vi "OverlayArcCenterSize.vi"(0 "Image Reference In":T3, 1 "GroupName":string, 2 "Start Angle (degrees)":dbl format="%.2f", 3 "End Angle (degrees)":dbl format="%.2f", 5 "Center-Point":T1, 7 "Size":T1, 11 "error in":errorcluster, 12 "Drawing Mode (Fill)":T2=enum."Fill", 13 "Color":u32(colorbox)=16711680) -> (4 "Image Reference Out":T3, 15 "error out":errorcluster)   [LabVIEW 2024, in "OpenLvVision_Overlays.lvlib"]
doc: "Overlay a arc on top of an image.\nDraws the arc arround a center point."
uses:
  OpenLvVision_Overlays.lvlib
  <vilib>/OpenLvVision/OpenLvVision_Image/Management/TypeDef/OLV Image.ctl
  TypeDefs/DrawingMode.ctl
  TypeDefs/PointI32.ctl
  <vilib>/OpenLvVision/OpenLvVision_Image/Management/OLV Management.lvlib
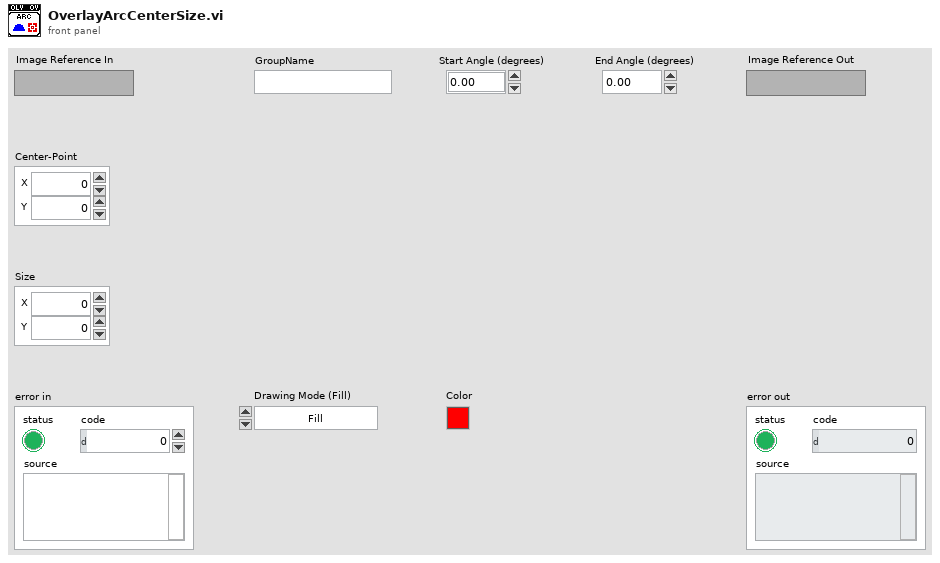
[diagram p1: front panel]
types:
  T1 = typedef "OpenLvVision_Overlays.lvlib/PointI32.ctl" = cluster{"X":i32, "Y":i32}
  T2 = typedef "OpenLvVision_Overlays.lvlib/DrawingMode.ctl" = enum16{"Frame", "Fill"}
  T3 = typedef "OLV OpenLvVision_Image.lvlib/OLV Management.lvlib/OLV Image.ctl" = refnum<image>
  T4 = typedef "OLV OpenLvVision_Image.lvlib/OLV DataAccess.lvlib/OLV RectangleI32.ctl" = cluster{"Left":i32, "Top":i32, "Right":i32, "Bottom":i32}
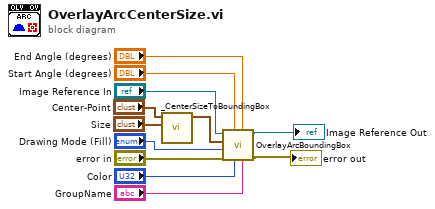
[diagram p0: block diagram]
diagram:
  n1 = call "_CenterSizeToBoundingBox.vi"("Size"="Size", "Center-Point"="Center-Point") -> ("Bounding Box"=w1:T4)  [unwired: 9 in]
  n2 = call "OverlayArcBoundingBox.vi"("GroupName"="GroupName", "End Angle (degrees)"="End Angle (degrees)", "Color"="Color", "Start Angle (degrees)"="Start Angle (degrees)", "error in"="error in", "Drawing Mode (Frame)"="Drawing Mode (Fill)", "BondingBox"=w1, "Image Reference In"="Image Reference In") -> ("error out"=→"error out":errorcluster, "Image Reference Out"=→"Image Reference Out":T3)  [unwired: 2 in]
